vi "ROIAndorNullValFGV.vi"(8 "error in":errorcluster, 10 "Set_Get":enum16{"Set", "Get"}(ring), 11 "set":bool=TRUE) -> (0 "error out":errorcluster, 3 "get":bool)   [LabVIEW 2011]
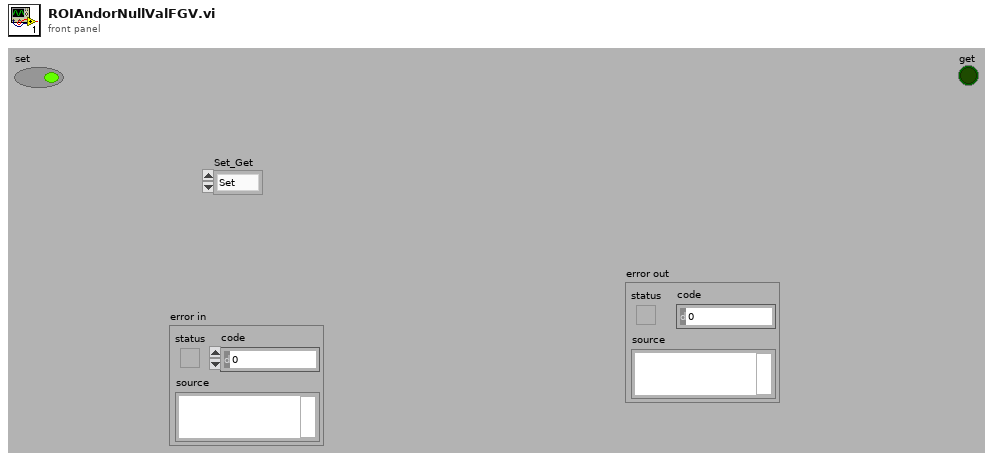
[diagram p1: front panel]
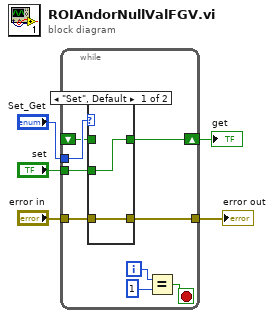
[diagram p0: block diagram]
diagram:
  n1 = while {
    tunnel: "Set_Get" -> [w14]
    tunnel: "set" -> [w13]
    shift-right: [w12] -> w1
    shift-left: _ -> [w11]
    tunnel: [w7] -> w4
    tunnel: "error in" -> [w6]
    i -> [w9]
    stop <- w10 stop-if-true
    n2 = case shown="\"Set\", Default" w14 {
      tunnel: w13 -> [w16 _]
      tunnel: [w16 w18] -> w12
      tunnel: w11 -> [_ w18]
      tunnel: [w15 w17] -> w7
      tunnel: w6 -> [w15 w17]
      frame "Set", Default {
      }
      frame "Get" {
      }
    }
    n3 = Equal?(x=w9, y=1) -> (x = y?=w10:bool)
  }
  "error out" <- w4
  "get" <- w1
